vi "MS SQL Day Report [tbl].vi"(0 "Ref In":T4={"MS SQL Connection"=refnum, "UDL File"=path "", "Time"="", "DCODE"="", "WIP+1"=0, "MC No?"=0, "POKAYOKE?"=FALSE, "Expected Result"="", "Result [Status]"="", "Clock"=0.0, "RFID"="", "WIP Queue"=refnum, "TS Parameter"={"ProfitCenterCode"="", "LineCode"="", "WorkOrderNumber"="", "Model"="", "Model_with_Prefix"="", "VendorCode"="", "SetParameterDateCode"="", "PokaYoke"=0, "Target"=1, "Live_DateCode"="", "CustomerPartNumber"="", "Hand"="", "Ent_Stamp"=timestamp(0 s since 1904-01-01), "sBarcode"=FALSE, "FCA"=0, "STS_CD"=0.0}, "Data_Queue"=[], "RFID Serial No."=""} {"TS Parameter"."FCA" format="%01d"; "TS Parameter"."Target" min=1 max=100000; "TS Parameter"."PokaYoke" min=0 max=1}, 1 "Report_Date":string, 2 "Filter In":T1[](array[typedef]), 3 "Audit":T3, 5 "RFID":string, 9 "Full Date?":bool=TRUE, 11 "error in (no error)":errorcluster, 12 "index":i32, 14 "Order By":i32) -> (4 "Report Data":string[][](array[string]), 6 "Column name":string[](array[string]), 10 "Lengths":i32[](array[numeric]), 15 "error out":errorcluster)   [LabVIEW 2020]
uses:
  Controls/TD SQL.ctl
  <vilib>/addons/database/Connection.llb/Conn ObjectReference.ctl
  Controls/WIP_State.ctl
  Controls/TS_Parameter.ctl
  <menus>/Controls/Devaseelan Style/ONOFF Small.ctl
  Controls/Filter.ctl
  Controls/Comparator.ctl
  <vilib>/addons/database/Auxilliary.llb/DB Tools DataTypes.ctl
  <userlib>/_OpenG.lib/comparison/comparison.llb/I32 Changed__ogtk.vi
  <userlib>/_OpenG.lib/array/array.llb/Search 1D Array (I32)__ogtk.vi
  <vilib>/addons/database/Connection.llb/Conn Execute.vi
  <vilib>/addons/database/Recordset.llb/Rec Fetch Recordset Data (R).vi
  <vilib>/addons/database/Recordset.llb/Rec Destroy - Connection.vi
  <vilib>/addons/database/NI_Database_API.lvlib
panel:
  out "resulting string":string
  out "deleted portion":string[][](array[string])
  out "recordset data":variant[][](array[variant])
  out "columns":string[](array[string])
  out "Changed":bool
  out "result string":string
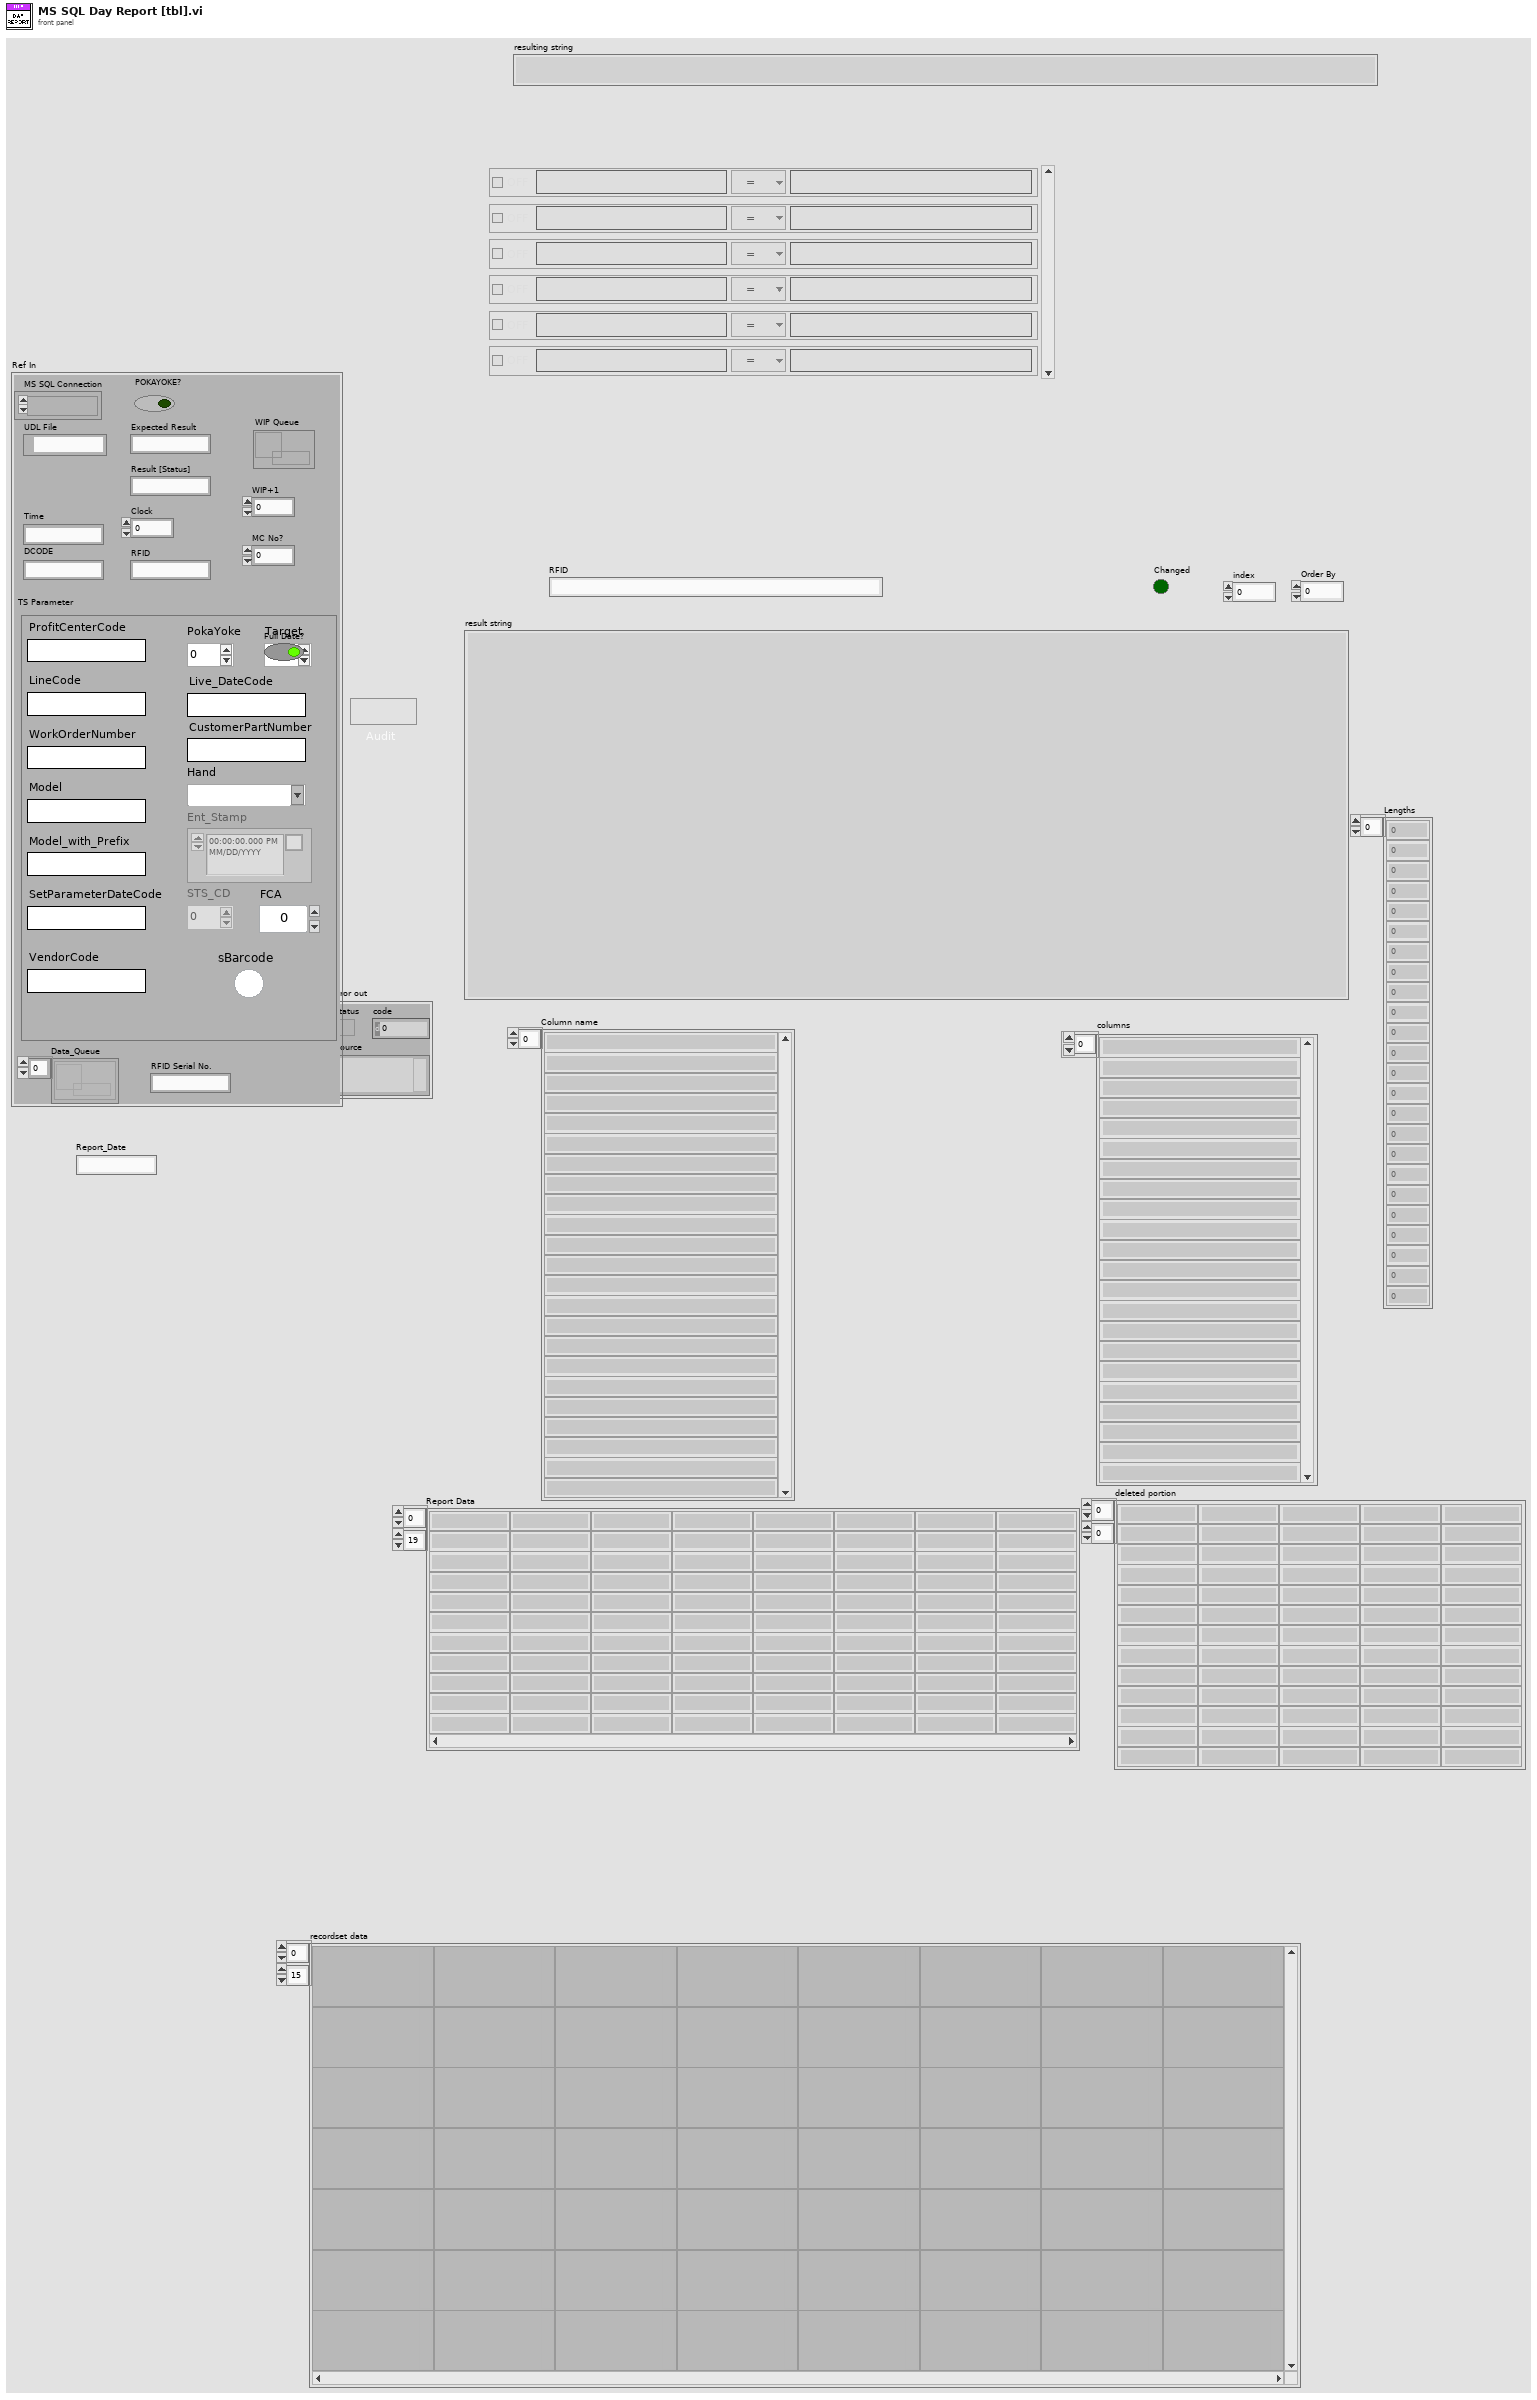
[diagram p1: front panel]
types:
  T1 = typedef "Filter.ctl" = cluster{"Select":bool, "Column":string, "Compare":T2, "Data":string}
  T2 = typedef "Comparator.ctl" = enum16{"=", "<=", ">=", "<", ">", "Like"}
  T3 = typedef "ONOFF Small.ctl" = bool
  T4 = typedef "TD SQL.ctl" = cluster{"MS SQL Connection":T5, "UDL File":path, "Time":string, "DCODE":string, "WIP+1":i64, "MC No?":i32, "POKAYOKE?":bool, "Expected Result":string, "Result [Status]":string, "Clock":dbl, "RFID":string, "WIP Queue":refnum<queue>, "TS Parameter":T6, "Data_Queue":refnum<queue>[], "RFID Serial No.":string}
  T5 = typedef "NI_Database_API.lvlib/Conn ObjectReference.ctl" = refnum<k1>
  T6 = typedef "TS_Parameter.ctl" = cluster{"ProfitCenterCode":string, "LineCode":string, "WorkOrderNumber":string, "Model":string, "Model_with_Prefix":string, "VendorCode":string, "SetParameterDateCode":string, "PokaYoke":i32, "Target":i32, "Live_DateCode":string, "CustomerPartNumber":string, "Hand":string, "Ent_Stamp":timestamp, "sBarcode":bool, "FCA":i32, "STS_CD":dbl}
  T7 = typedef "NI_Database_API.lvlib/DB Tools DataTypes.ctl" = enum16{"String", "Long (I32)", "Single (SGL)", "Double (DBL)", "Date/Time", "Binary"}
  T8 = cluster{"name":string, "database data type":T7, "defined size":i32}[]
  T9 = typedef "NI_Database_API.lvlib/Rec ObjectReference.ctl" = refnum<k1>
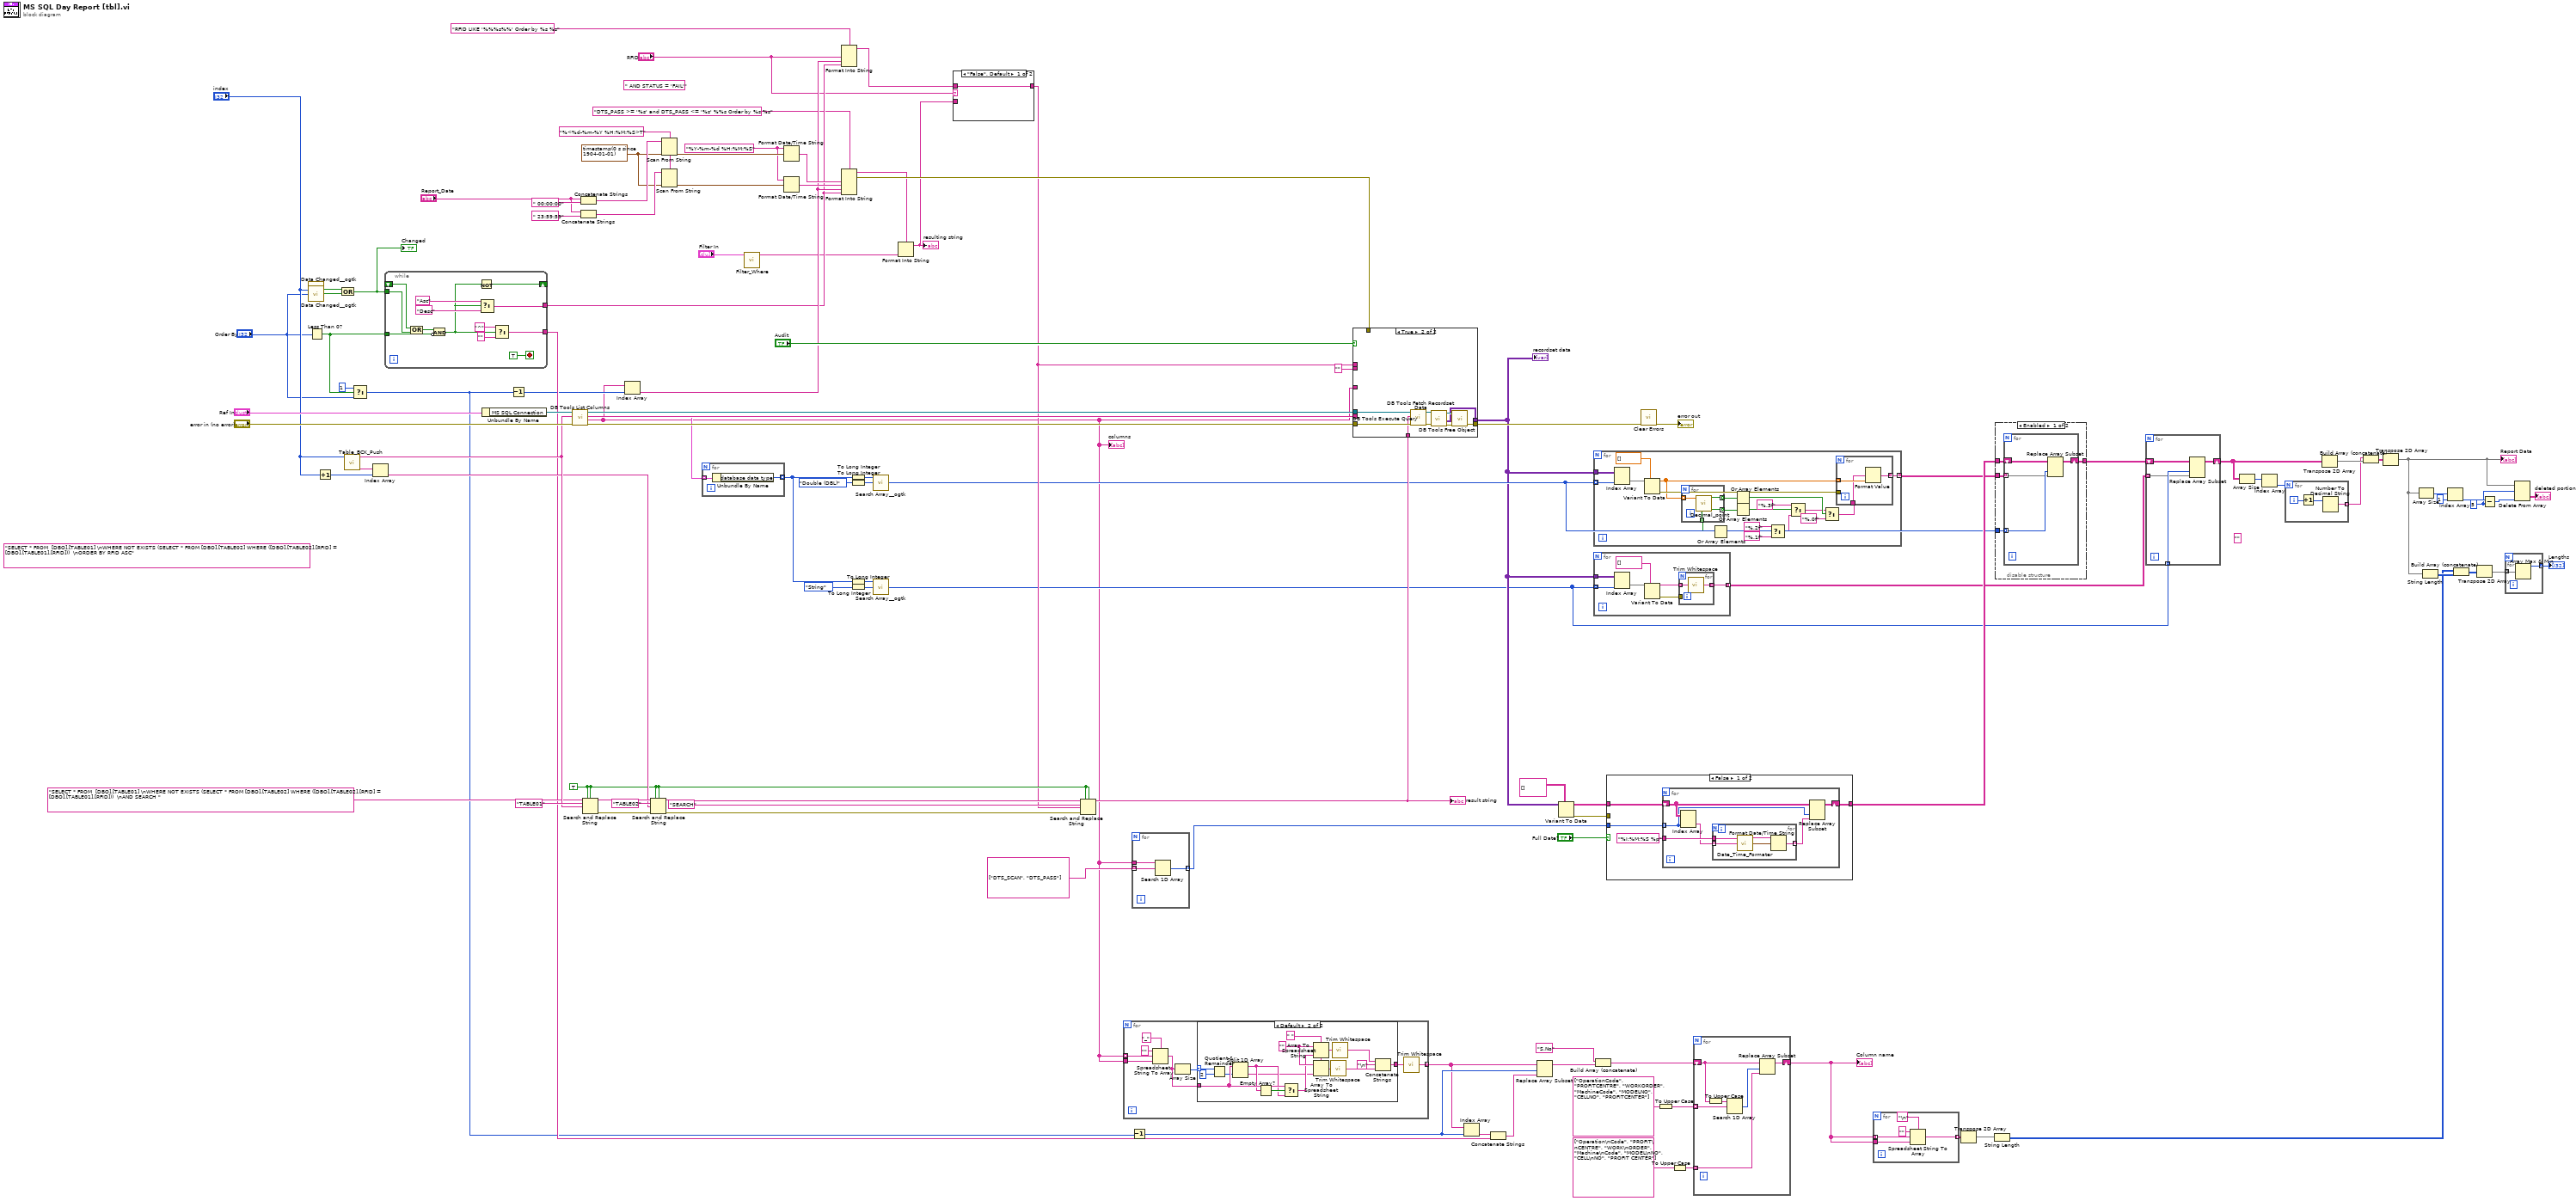
[diagram p0: block diagram]
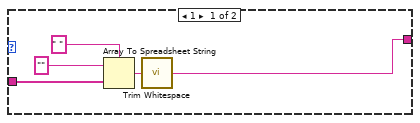
[diagram p2: hidden frame]
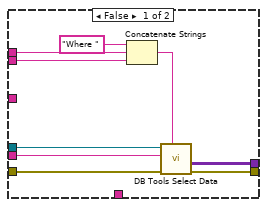
[diagram p6: hidden frame]
diagram:
  w25 = 5 ("y")
  (unwired) "" ("table")
  (unwired) " AND STATUS = 'FAIL'" ("string")
  w76 = TRUE ("replace all? (F)")
  (unwired) "SELECT * FROM  [DBO].[TABLE01] \nWHERE NOT EXISTS (SELECT * FROM [DBO].[TABLE02] WHERE ([DBO].[TABLE02].[RFID] = [DBO].[TABLE01].[RFID]))  \nORDER BY RFID ASC"
  w103 = "%Y-%m-%d %H:%M:%S" ("time format string (%c)")
  w109 = "%<%d-%m-%Y %H:%M:%S>T" ("time format string (%c)")
  w106 = timestamp(0 s since 1904-01-01) ("time stamp")
  n1 = call-poly <userlib>:"Data Changed__ogtk.vi"("I32"="index") -> ("Changed"=w54:bool)
  n2 = call-poly <userlib>:"Data Changed__ogtk.vi"("I32"="Order By") -> ("Changed"=w65:bool)
  n3 = Less Than 0?(x="Order By") -> (x < 0?=w18:bool)
  n4 = Increment(x="index") -> (x+1=w78:i32)
  n5 = Compound Arithmetic op=OR(w54, w65) -> (w56:bool)
  "Changed" <- w56
  n6 = call "Table_BCK_Push.vi"("index"="index") -> ("Tables[]"=w79:string[], "Table Name"=w80:string)  [unwired: 9 in]
  n7 = Select(t=1, s=w18, f="Order By") -> (s? t:f=w16:i32)
  n8 = Index Array(array=w79, index=w78) -> (element=w77:string)
  n9 = while {
    tunnel: w56 -> [w120]
    shift-right: [w118] -> _
    shift-left: _ -> [w119]
    tunnel: [w122] -> w59
    tunnel: [w115] -> w63
    tunnel: w18 -> [w113]
    stop <- TRUE stop-if-true
    n10 = Compound Arithmetic op=OR(w119, w120) -> (w114:bool)
    n11 = Compound Arithmetic op=AND(w114, invert w113) -> (w112:bool)
    n12 = Not(x=w112) -> (.not. x?=w118:bool)
    n13 = Select(t="Asc" ("time format string (%c)"), s=w112, f="Desc") -> (s? t:f=w122:string)
    n14 = Select(t="^" ("f"), s=w112, f="") -> (s? t:f=w115:string)
  }
  n15 = Unbundle By Name("Ref In") -> ("MS SQL Connection"=w90:T5)
  n16 = Decrement(x=w16) -> (x-1=w62:i32)
  n17 = call <vilib>:"DB Tools List Columns.vi"("error in (no error)"="error in (no error)", "table"=w80, "connection reference"=w90) -> ("error out"=w87:errorcluster, "columns"=w2:string[], "column information"=w45:T8, "connection reference out"=w89:T5)  [unwired: 1 in]
  "columns" <- w2
  n18 = Concatenate Strings("Report_Date", " 00:00:00" ("time format string (%c)")) -> (w108:string)
  n19 = Concatenate Strings("Report_Date", " 23:59:59" ("time format string (%c)")) -> (w107:string)
  n20 = Search and Replace String(replace all?=w76, case sensitive?=w76, input string="SELECT * FROM  [DBO].[TABLE01] \nWHERE NOT EXISTS (SELECT * FROM [DBO].[TABLE02] WHERE ([DBO].[TABLE02].[RFID] = [DBO].[TABLE01].[RFID]))  \nAND SEARCH ", search string="TABLE01", replace string=w80) -> (result string=w83:string, error out=w75:errorcluster)  [unwired: 3 in, 2 out]
  n21 = Index Array(array=w2, index=w62) -> (element=w60:string)
  n22 = Search and Replace String(replace all?=w76, case sensitive?=w76, input string=w83, search string="TABLE02", replace string=w77, error in=w75) -> (result string=w82:string, error out=w74:errorcluster)  [unwired: 2 in, 2 out]
  n23 = Scan From String(format string=w109, input string=w108, default 1=w106) -> (output 1=w105:timestamp)  [unwired: 2 in, 3 out]
  n24 = Scan From String(format string=w109, input string=w107, default 1=w106) -> (output 1=w102:timestamp)  [unwired: 2 in, 3 out]
  n25 = for {
    tunnel: w45 -> [w126] mode=indexing
    tunnel: [w125] -> w35 mode=indexing
    n26 = Unbundle By Name(w126) -> ("database data type"=w125:T7)
  }
  n27 = call "Filter_Where.vi"("Filter In"="Filter In") -> ("WHERE?"=w22:string)  [unwired: 10 in]
  n28 = Format Date/Time String(time format string (%c)=w103, seconds (now)=w105) -> (date/time string=w104:string)  [unwired: 1 in]
  n29 = Format Date/Time String(time format string (%c)=w103, seconds (now)=w102) -> (date/time string=w101:string)  [unwired: 1 in]
  n30 = Format Into String(format string="RFID LIKE '%%%s%%' Order by %s %s" ("time format string (%c)"), "RFID", w60, w59) -> (resulting string=w57:string)  [unwired: 2 in, 1 out]
  n31 = Format Into String(format string="DTS_PASS >= '%s' and DTS_PASS <= '%s' %%s Order by %s %s" ("resulting string 2"), w104, w101, w60, w59) -> (resulting string=w20:string, error out=w64:errorcluster)  [unwired: 2 in]
  n32 = To Long Integer(number=w35) -> (32bit integer=w44:i32[])
  n33 = To Long Integer(number=DB_Tools_DataTypes."Double (DBL)" ("database data type")) -> (32bit integer=w42:i32)
  n34 = To Long Integer(number=w35) -> (32bit integer=w36:i32[])
  n35 = To Long Integer(number=DB_Tools_DataTypes."String" ("database data type")) -> (32bit integer=w38:i32)
  n36 = call-poly <userlib>:"Search Array__ogtk.vi"("Array"=w44, "Element Data"=w42) -> ("Indices of Elements"=w40:i32[])  [unwired: 7 in]
  n37 = call-poly <userlib>:"Search Array__ogtk.vi"("Array"=w36, "Element Data"=w38) -> ("Indices of Elements"=w31:i32[])  [unwired: 7 in]
  n38 = Format Into String(format string=w20, w22) -> (resulting string=w19:string)  [unwired: 2 in, 1 out]
  "resulting string" <- w19
  n39 = case shown="\"False\", Default" "RFID" {
    tunnel: w19 -> [_ w128]
    tunnel: w57 -> [w127 _]
    tunnel: [w127 w128] -> w48
    frame "False", Default {
    }
    frame "--" {
    }
  }
  n40 = Search and Replace String(replace all?=w76, case sensitive?=w76, input string=w82, search string="SEARCH", replace string=w48, error in=w74) -> (result string=w72:string)  [unwired: 2 in, 3 out]
  "result string" <- w72
  n41 = for {
    tunnel: w2 -> [w136] mode=indexing
    tunnel: [w131] -> w1 mode=indexing
    tunnel: w2 -> [w133]
    n42 = Spreadsheet String To Array(delimiter (Tab)="_" ("search string"), format string="", spreadsheet string=w136, array type (2D Dbl)=w133) -> (array=w130:string[])
    n43 = Array Size(array=w130) -> (size(s)=w129:i32)
    n44 = case shown="Default" w129 {
      selector: w129 -> [_ w142]
      tunnel: [w137 w152] -> w132
      tunnel: w130 -> [w138 w147]
      frame 1 {
        n45 = Array To Spreadsheet String(delimiter (Tab)=" ", array=w138, 3:"" ("format string")) -> (spreadsheet string=w139:string)
        n46 = call <vilib>:"Trim Whitespace.vi"("string"=w139) -> ("trimmed string"=w137:string)  [unwired: 1 in]
      }
      frame Default {
        w157 = " " ("delimiter (Tab)")
        w156 = "" ("format string")
        n47 = Quotient & Remainder(x=w142, y=2) -> (floor(x/y)=w143:i32)  [unwired: 1 out]
        n48 = Split 1D Array(array=w147, index=w143) -> (first subarray=w145:string[], second subarray=w144:string[])
        n49 = Empty Array?(array=w145) -> (empty?=w149:bool)
        n50 = Select(t=w147, s=w149, f=w145) -> (s? t:f=w148:string[])
        n51 = Array To Spreadsheet String(delimiter (Tab)=w157, array=w148, 3:w156) -> (spreadsheet string=w155:string)
        n52 = Array To Spreadsheet String(delimiter (Tab)=w157, array=w144, 3:w156) -> (spreadsheet string=w154:string)
        n53 = call <vilib>:"Trim Whitespace.vi"("string"=w154) -> ("trimmed string"=w150:string)  [unwired: 1 in]
        n54 = call <vilib>:"Trim Whitespace.vi"("string"=w155) -> ("trimmed string"=w151:string)  [unwired: 1 in]
        n55 = Concatenate Strings(w151, "\n" ("format string"), w150) -> (w152:string)
      }
    }
    n56 = call <vilib>:"Trim Whitespace.vi"("string"=w132) -> ("trimmed string"=w131:string)  [unwired: 1 in]
  }
  n57 = Decrement(x=w16) -> (x-1=w66:i32)
  n58 = for {
    tunnel: w2 -> [w160]
    tunnel: string[] ["DTS_SCAN", "DTS_PASS"] ("output array") -> [w159] mode=indexing
    tunnel: [w158] -> w49 mode=indexing
    n59 = Search 1D Array(1D array=w160, element=w159) -> (index of element=w158:i32)  [unwired: 1 in]
  }
  n60 = case shown="True" "Audit" {
    tunnel: [w169 w171] -> w34
    tunnel: [w168 w170] -> w99
    tunnel: w89 -> [w167 w174]
    tunnel: w87 -> [w166 w173]
    tunnel: w80 -> [w165 _]
    tunnel: w48 -> [w164 _]
    tunnel: w72 -> [_ w172]
    tunnel: "" ("time format string (%c)") -> [w161 _]
    tunnel: w64 -> [_ _]
    tunnel: w2 -> [_ _]
    frame False {
      n61 = Concatenate Strings("Where " ("time format string (%c)"), w164, w161) -> (w163:string)
      n62 = call <vilib>:"DB Tools Select Data.vi"("condition"=w163, "error in (no error)"=w166, "table"=w165, "connection reference"=w167) -> ("error out"=w168:errorcluster, "data"=w169:variant[][])  [unwired: 2 in, 1 out]
    }
    frame True {
      n63 = call-poly <vilib>:"DB Tools Execute Query.vi"("error in (no error)"=w173, "SQL query"=w172, "connection reference"=w174) -> ("error out"=w178:errorcluster, "recordset reference"=w177:T9)  [unwired: 5 in]
      n64 = call-poly <vilib>:"DB Tools Fetch Recordset Data.vi"("error in (no error)"=w178, "recordset reference"=w177) -> ("error out"=w175:errorcluster, "recordset data"=w171:variant[][], "recordset reference out"=w176:T9)  [unwired: 3 in]
      n65 = call-poly <vilib>:"DB Tools Free Object.vi"("error in (no error)"=w175, "recordset reference"=w176) -> ("error out"=w170:errorcluster)  [unwired: 8 in, 1 out]
    }
  }
  "recordset data" <- w34
  n66 = Index Array(array=w1, index=w66) -> (element=w69:string)
  n67 = Concatenate Strings(w69, w63) -> (w68:string)
  n68 = Replace Array Subset(array=w1, new element=w68, index=w66) -> (w67:string[])
  n69 = Variant To Data(type=string[][] [], Variant=w34) -> (data=w50:string[][], error out=w47:errorcluster)  [unwired: 1 in]
  n70 = for {
    tunnel: w34 -> [w198]
    tunnel: w40 -> [w197] mode=indexing
    tunnel: [w194] -> w39 mode=indexing
    n71 = Index Array(array=w198, index (col)=w197) -> (element=w196:variant[])  [unwired: 1 in]
    n72 = Variant To Data(type=dbl[] [], Variant=w196) -> (data=w192:dbl[], error out=w193:errorcluster)  [unwired: 1 in]
    n73 = for {
      tunnel: w192 -> [w202] mode=indexing
      tunnel: [w201] -> w191 mode=indexing
      tunnel: [w200] -> w190 mode=indexing
      tunnel: [w199] -> w183 mode=indexing
      n74 = call "Decimal_point.vi"("Numeric"=w202) -> ("2|3?"=w200:bool, "Decimal?"=w201:bool, "1|2?"=w199:bool)  [unwired: 8 in]
    }
    n75 = Or Array Elements(Boolean array=w183) -> (logical OR=w180:bool)
    n76 = Or Array Elements(Boolean array=w191) -> (logical OR=w187:bool)
    n77 = Or Array Elements(Boolean array=w190) -> (logical OR=w189:bool)
    n78 = Select(t="%.2f" ("format string"), s=w180, f="%.1f" ("format string")) -> (s? t:f=w179:string)
    n79 = Select(t="%.3f" ("format string"), s=w189, f=w179) -> (s? t:f=w186:string)
    n80 = Select(t=w186, s=w187, f="%.0f" ("format string")) -> (s? t:f=w184:string)
    n81 = for {
      tunnel: w192 -> [w205] mode=indexing
      tunnel: [w204] -> w194 mode=indexing
      tunnel: w193 -> [_]
      tunnel: w184 -> [w203]
      n82 = Format Value(format string=w203, value (0)=w205) -> (output string=w204:string)  [unwired: 1 in]
    }
  }
  n83 = for {
    tunnel: w34 -> [w212]
    tunnel: w31 -> [w211] mode=indexing
    tunnel: [w206] -> w32 mode=indexing
    n84 = Index Array(array=w212, index (col)=w211) -> (element=w210:variant[])  [unwired: 1 in]
    n85 = Variant To Data(type=string[] [], Variant=w210) -> (data=w207:string[], error out=w208:errorcluster)  [unwired: 1 in]
    n86 = for {
      tunnel: w208 -> [_]
      tunnel: w207 -> [w214] mode=indexing
      tunnel: [w213] -> w206 mode=indexing
      n87 = call <vilib>:"Trim Whitespace.vi"("string"=w214) -> ("trimmed string"=w213:string)  [unwired: 1 in]
    }
  }
  n88 = Build Array (concatenate)("S.No" ("result string"), w67) -> (w4:string[])
  n89 = case shown="False" "Full Date?" {
    tunnel: w50 -> [w218 w229]
    tunnel: w49 -> [w217 _]
    tunnel: [w215 w229] -> w41
    tunnel: w47 -> [_ _]
    frame False {
      n90 = for {
        tunnel: w217 -> [w221] mode=indexing
        tunnel: "%I:%M:%S %p" ("time format string (%c)") -> [w224]
        shift-right: [w219] -> w215
        shift-left: w218 -> [w222]
        n91 = Index Array(array=w222, index (col)=w221) -> (element=w223:string[])  [unwired: 1 in]
        n92 = for {
          tunnel: w224 -> [w228]
          tunnel: w223 -> [w226] mode=indexing
          tunnel: [w227] -> w220 mode=indexing
          n93 = call "Date_Time_Formater.vi"("Date In"=w226) -> ("Date Out"=w225:timestamp)
          n94 = Format Date/Time String(time format string (%c)=w228, seconds (now)=w225) -> (date/time string=w227:string)  [unwired: 1 in]
        }
        n95 = Replace Array Subset(array=w222, new element=w220, index (col)=w221) -> (w219:string[][])  [unwired: 1 in]
      }
    }
    frame True {
    }
  }
  n96 = call <vilib>:"Clear Errors.vi"("error in (no error)"=w99) -> ("error out"=→"error out":errorcluster)  [unwired: 5 in, 1 out]
  n97 = To Upper Case(1:string[] ["OperationCode", "PROFITCENTRE", "WORKORDER", "MachineCode", "MODELNO", "CELLNO", "PROFITCENTER"] ("output array")) -> (0:w5:string[])
  n98 = To Upper Case(1:string[] ["Operation\nCode", "PROFIT\nCENTRE", "WORK\nORDER", "Machine\nCode", "MODEL\nNO", "CELL\nNO", "PROFIT CENTER"] ("output array")) -> (0:w14:string[])
  n99 = for {
    shift-right: [w232] -> w3
    shift-left: w4 -> [w235]
    tunnel: w5 -> [w230] mode=indexing
    tunnel: w14 -> [w233] mode=indexing
    n100 = To Upper Case(1:w235) -> (0:w231:string[])
    n101 = Search 1D Array(1D array=w231, element=w230) -> (index of element=w234:i32)  [unwired: 1 in]
    n102 = Replace Array Subset(array=w235, new element=w233, index=w234) -> (w232:string[])
  }
  "Column name" <- w3
  n103 = for {
    tunnel: w3 -> [w240] mode=indexing
    tunnel: w3 -> [w237]
    tunnel: [w236] -> w13 mode=indexing
    n104 = Spreadsheet String To Array(delimiter (Tab)="\n", format string="", spreadsheet string=w240, array type (2D Dbl)=w237) -> (array=w236:string[])
  }
  n105 = Transpose 2D Array(2D array=w13) -> (transposed array=w10:string[][])
  n106 = String Length(string=w10) -> (length=w11:i32[][])
  n107 = disable-structure shown="Enabled" {
    disable-tunnel: w41 -> [w244 w249]
    disable-tunnel: w40 -> [w243 _]
    disable-tunnel: w39 -> [w242 _]
    disable-tunnel: [w241 w249] -> w33
    frame Enabled {
      n108 = for {
        shift-right: [w245] -> w241
        shift-left: w244 -> [w248]
        tunnel: w243 -> [w247] mode=indexing
        tunnel: w242 -> [w246] mode=indexing
        n109 = Replace Array Subset(array=w248, new element=w246, index (col)=w247) -> (w245:string[][])  [unwired: 1 in]
      }
    }
    frame Disabled {
    }
  }
  n110 = for {
    shift-right: [w250] -> w30
    shift-left: w33 -> [w253]
    tunnel: w31 -> [w252] mode=indexing
    tunnel: w32 -> [w251] mode=indexing
    n111 = Replace Array Subset(array=w253, new element=w251, index (col)=w252) -> (w250:string[][])  [unwired: 1 in]
  }
  n112 = Array Size(array=w30) -> (size(s)=w95:i32[])
  n113 = Index Array(array=w95) -> (element=w94:i32)  [unwired: 1 in]
  n114 = for {
    N: w94 -> [_]
    tunnel: [w254] -> w91 mode=indexing
    i -> [w256]
    n115 = Increment(x=w256) -> (x+1=w255:i32)
    n116 = Number To Decimal String(number=w255) -> (decimal integer string=w254:string)  [unwired: 1 in]
  }
  n117 = Transpose 2D Array(2D array=w30) -> (transposed array=w92:string[][])
  n118 = Build Array (concatenate)(w91, w92) -> (w93:string[][])
  n119 = Transpose 2D Array(2D array=w93) -> (transposed array=w6:string[][])
  "Report Data" <- w6
  n120 = Array Size(array=w6) -> (size(s)=w29:i32[])
  n121 = String Length(string=w6) -> (length=w12:i32[][])
  n122 = Index Array(array=w29, index=1) -> (element=w27:i32)
  n123 = Build Array (concatenate)(w11, w12) -> (w9:i32[][])
  n124 = Transpose 2D Array(2D array=w9) -> (transposed array=w8:i32[][])
  n125 = Subtract(x=w27, y=w25) -> (x-y=w26:i32)
  n126 = for {
    tunnel: w8 -> [w258] mode=indexing
    tunnel: [w257] -> w7 mode=indexing
    n127 = Array Max & Min(array=w258) -> (max value=w257:i32)  [unwired: 3 out]
  }
  "Lengths" <- w7
  n128 = Delete From Array(array=w6, length=w25, index (col)=w26) -> (deleted portion=→"deleted portion":string[][])  [unwired: 1 in, 1 out]
